vi "Encode-Decode Parameters (core).vi"(9 "Payload size - bytes":i32=16, 10 "Parameters":T2(array[cluster])=[{"start index"=0, "size"=64, "encoding"=0, "signed"=TRUE, "scale multiplier"=1.0, "scale offset"=0.0}, {"start index"=64, "size"=64, "encoding"=0, "signed"=TRUE, "scale multiplier"=1.0, "scale offset"=0.0}] {"encoding" items=["BNR", "BCD", "Discrete", "Signed_32", "Signed_64", "Float_32", "Float_64", "Opaque"]}, 11 "Values in":dbl[](array[numeric])) -> (2 "Result array out":bool[](array[boolean]), 3 "Values out":dbl[](array[numeric]))   [LabVIEW 2020, in "AIM ARINC 664 EncodeDecode.lvclass"]
uses:
  AIM ARINC 664 EncodeDecode.lvclass
  Shared/Encoding (Arinc664).ctl
  Shared/Encode Payload Data from Channels.vi/b24d3698-aaae-4200-bf93-4b6af5480478.vi
  Shared/Encode Payload Data from Channels.vi/5b1080be-549e-4688-aad8-fb955257d8ef.vi
  Shared/Encode Payload Data from Channels.vi/2afa5e5b-ae47-4ac6-b34f-e51087edfaba.vi
  Shared/Convert U8 Array to Bool Array.vi
  Shared/Encode Payload Data from Channels.vi/1eaed3cb-9180-4944-bca4-c812fd7aad88.vi
  Shared/Encode Payload Data from Channels.vi/f46899e6-f3c2-4da0-acc2-ed34a334556c.vi
  Shared/Encode Payload Data from Channels.vi/7b487445-4b60-493e-9c15-0f5b7677c2b1.vi
  Shared/Encode Payload Data from Channels.vi/7e7e8f0d-6015-4215-b4f4-37ecf7ce16f3.vi
  Shared/Convert bool array to U8 Array.vi
  Shared/Encode Payload Data from Channels.vi/b24d3698-aaae-4200-bf93-4b6af5480478.vi/9377bb8f-44b5-4a8f-87f1-966fd5a9edcc.vi
  Shared/Encode Payload Data from Channels.vi/b24d3698-aaae-4200-bf93-4b6af5480478.vi/e95d9d1f-307c-44d6-9f26-c3f519a4990d.vi
  Shared/Encode Payload Data from Channels.vi/b24d3698-aaae-4200-bf93-4b6af5480478.vi/0c23f515-4369-4514-bc3d-4444e6b437b2.vi
  Shared/Encode Payload Data from Channels.vi/5b1080be-549e-4688-aad8-fb955257d8ef.vi/136dcdcb-2dd3-4a4d-a796-a8f7a3f8e1ac.vi
  Shared/Encode Payload Data from Channels.vi/5b1080be-549e-4688-aad8-fb955257d8ef.vi/a54b505c-1216-4ef4-8378-3ceda9d188df.vi
  <vilib>/NI/NI VeriStand Encoding and Decoding/Get Bits Per Digit from Base.vi
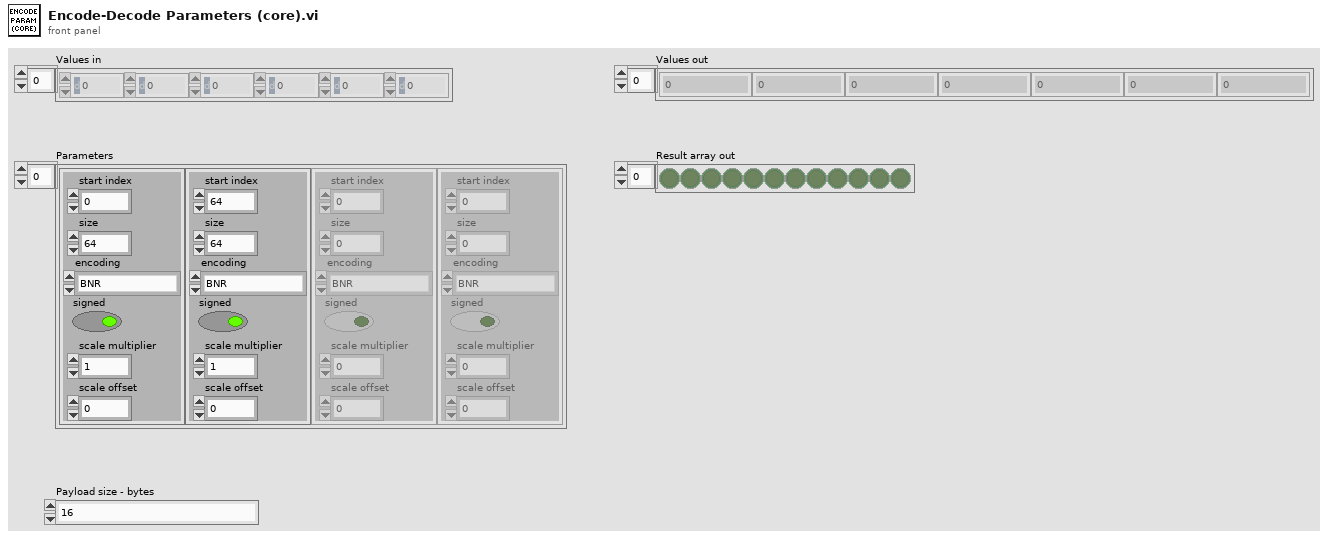
[diagram p1: front panel]
types:
  T1 = typedef "Encoding (Arinc664).ctl" = u16
  T2 = cluster{"start index":i32, "size":i32, "encoding":T1, "signed":bool, "scale multiplier":dbl, "scale offset":dbl}[]
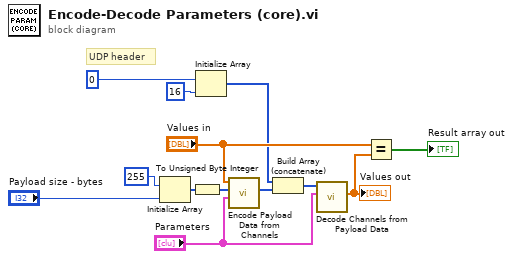
[diagram p0: block diagram]
diagram:
  # "UDP header"
  n1 = Initialize Array(255 ("dimension size"), "Payload size - bytes") -> (w11:i32[])
  n2 = To Unsigned Byte Integer(number=w11) -> (unsigned 8bit integer=w1:u8[])
  n3 = Initialize Array(u8 0 ("element"), 16 ("dimension size")) -> (w6:u8[])
  n4 = call "Encode Payload Data from Channels.vi"("Parameters"="Parameters", "Data in"=w1, "Values in"="Values in") -> ("Data out"=w3:u8[])  [unwired: 6 in, 2 out]
  n5 = Build Array (concatenate)(w6, w3) -> (w2:u8[])
  n6 = call "Decode Channels from Payload Data.vi"("Parameters"="Parameters", "Message Buffer in"=w2) -> ("Channels"=w8:dbl[])  [unwired: 8 in, 1 out]
  "Values out" <- w8
  n7 = Equal?(x="Values in", y=w8) -> (x = y?=→"Result array out":bool[])
